vi "Temp subvi.vi"(9 "y":dbl, 10 "y 2":dbl, 11 "Slide":dbl) -> (3 "Numeric":dbl)   [LabVIEW 2018]
panel:
  in  "Boolean":bool
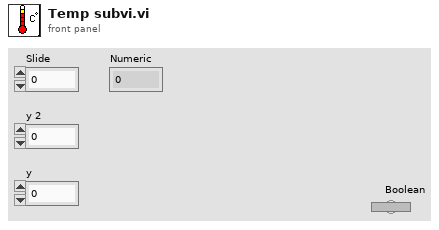
[diagram p1: front panel]
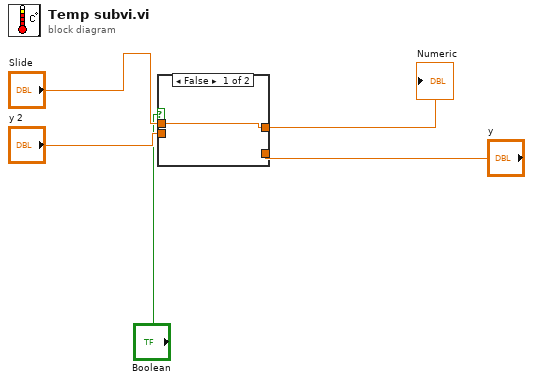
[diagram p0: block diagram]
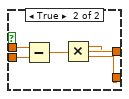
[diagram p2: hidden frame]
diagram:
  n1 = case shown="False" "Boolean" {
    tunnel: [w6 w11] -> w5
    tunnel: "y" -> [_ w9]
    tunnel: "Slide" -> [w6 w8]
    tunnel: "y 2" -> [_ w7]
    frame False {
    }
    frame True {
      n2 = Subtract(x=w8, y=w7) -> (x-y=w10:dbl)
      n3 = Multiply(x=w10, y=w9) -> (x*y=w11:dbl)
    }
  }
  "Numeric" <- w5
